vi "~pseudocode.vi"   [LabVIEW 2017]
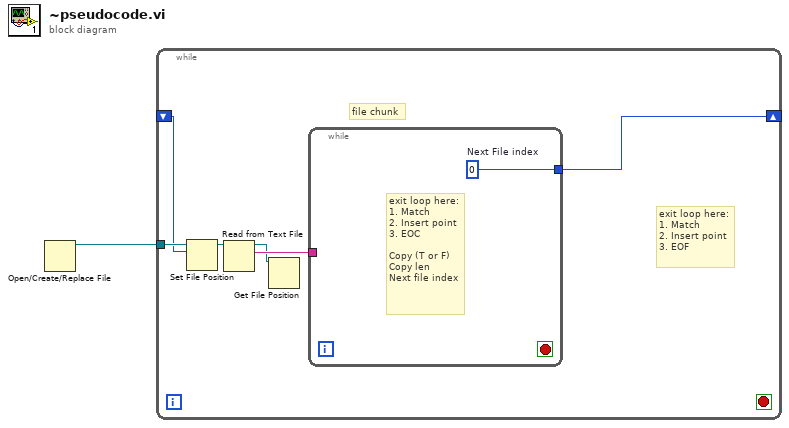
[diagram p0: block diagram]
diagram:
  n1 = Open/Create/Replace File() -> (refnum out=w1:refnum<file>)  [unwired: 6 in, 2 out]
  n2 = while {
    shift-right: [w4] -> _
    shift-left: _ -> [w2]
    tunnel: w1 -> [w6]
    stop <- _ stop-if-true
    # "file chunk"
    # "exit loop here:\n1. Match\n2. Insert point\n3. EOF"
    n3 = Set File Position(offset (in bytes) (0)=w2) -> ()  [unwired: 3 in, 2 out]
    n4 = Read from Text File(file (use dialog)=w6) -> (refnum out=w3:refnum<file>, text=w5:string)  [unwired: 3 in, 2 out]
    n5 = Get File Position(7:w3) -> ()  [unwired: 1 in, 3 out]
    n6 = while {
      tunnel: w5 -> [_]
      tunnel: [w7] -> w4
      stop <- _ stop-if-true
      w7 = i64 0  # Next File index
      # "exit loop here:\n1. Match\n2. Insert point\n3. EOC\n\nCopy (T or F)\nCopy len\nNext file index"
    }
  }
